vi "Clousure.vi"(8 "error in (no error)":errorcluster, 11 "ChicagoPizzaStore":refnum<class "ChicagoPizzaStore.lvclass">) -> (0 "error out":errorcluster, 3 "ChicagoPizzaStore":refnum<class "ChicagoPizzaStore.lvclass">)   [LabVIEW 2020, in "FactoryMethod.lvlib" / "PizzaFactoryMethod.lvlib" / "ChicagoPizzaStore.lvclass"]
uses:
  ChicagoPizzaStore.lvclass
  PizzaStore/PizzaStore.lvclass
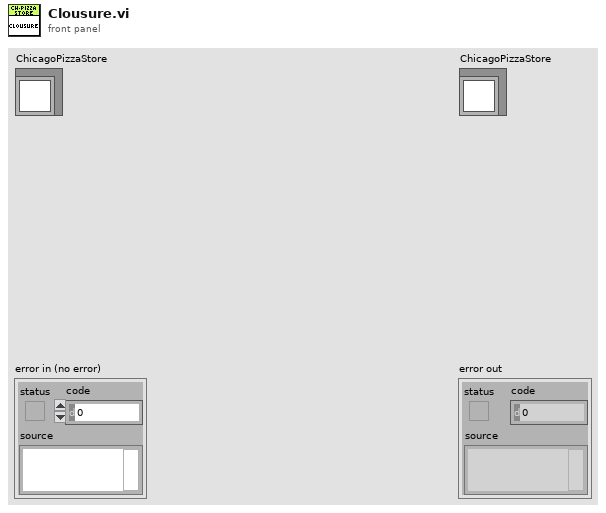
[diagram p1: front panel]
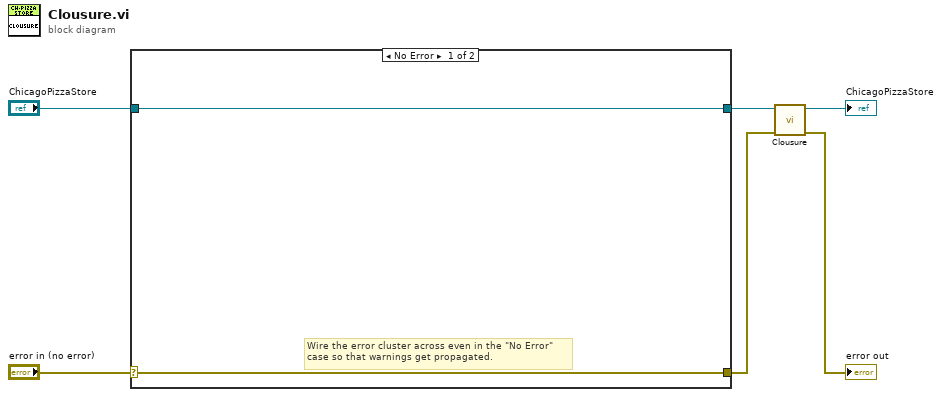
[diagram p0: block diagram]
diagram:
  n1 = case shown="No Error" "error in (no error)" {
    selector: "error in (no error)" -> [w7 w10]
    tunnel: [w7 w10] -> w2
    tunnel: [w8 w9] -> w4
    tunnel: "ChicagoPizzaStore" -> [w8 w9]
    frame No Error {
      # "Wire the error cluster across even in the \"No Error\"\ncase so that warnings get propagated."
    }
    frame Error {
    }
  }
  n2 = call-parent "Clousure.vi"("error in (no error)"=w2, "PizzaStore"=w4) -> ("error out"=→"error out":errorcluster, "PizzaStore"=→"ChicagoPizzaStore":refnum<class "ChicagoPizzaStore.lvclass">)  [unwired: 8 in]
